vi "Split Start Delays.vi"(0 "Start Delay":dbl, 5 "Value":dbl, 7 "Sequence Delta (s)":dbl) -> (4 "Start Delay":dbl[](array[numeric]), 6 "Value":dbl[](array[numeric]))   [LabVIEW 2024, in "devicePowerSequencerCoreLogic.lvlib"]
uses:
  devicePowerSequencerCoreLogic.lvlib
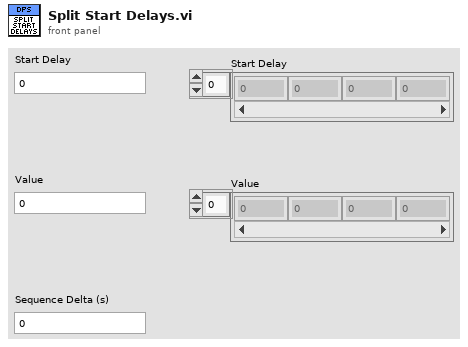
[diagram p1: front panel]
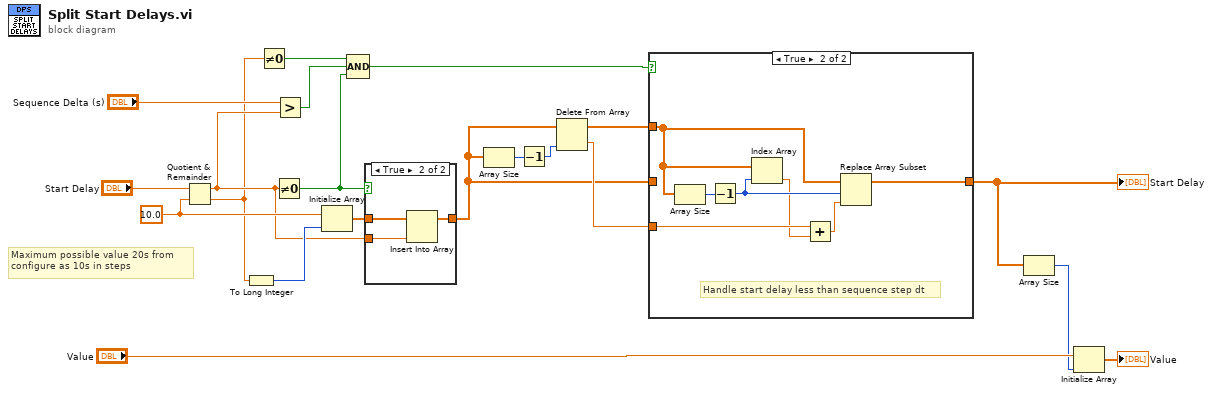
[diagram p0: block diagram]
diagram:
  w20 = 10.0 ("y")
  # "Maximum possible value 20s from\nconfigure as 10s in steps"
  n1 = Quotient & Remainder(x="Start Delay", y=w20) -> (x-y*floor(x/y)=w6:dbl, floor(x/y)=w5:dbl)
  n2 = To Long Integer(number=w5) -> (32bit integer=w18:i32)
  n3 = Not Equal To 0?(x=w5) -> (x != 0?=w4:bool)
  n4 = Not Equal To 0?(x=w6) -> (x != 0?=w2:bool)
  n5 = Greater?(x="Sequence Delta (s)", y=w6) -> (0:w3:bool)
  n6 = Initialize Array(w20, w18) -> (w19:dbl[])
  n7 = Compound Arithmetic op=AND(w4, w3, w2) -> (w1:bool)
  n8 = case shown="True" w2 {
    tunnel: w19 -> [w21 w24]
    tunnel: [w21 w22] -> w9
    tunnel: w6 -> [_ w23]
    frame False {
    }
    frame True {
      n9 = Insert Into Array(array=w24, new element=w23) -> (w22:dbl[])  [unwired: 1 in]
    }
  }
  n10 = Array Size(array=w9) -> (size(s)=w16:i32)
  n11 = Decrement(x=w16) -> (x-1=w15:i32)
  n12 = Delete From Array(array=w9, index=w15) -> (deleted portion=w13:dbl, array with subset deleted=w12:dbl[])  [unwired: 1 in]
  n13 = case shown="True" w1 {
    tunnel: w13 -> [_ w31]
    tunnel: [w25 w29] -> w8
    tunnel: w12 -> [_ w27]
    tunnel: w9 -> [w25 _]
    frame False {
    }
    frame True {
      # "Handle start delay less than sequence step dt"
      n14 = Array Size(array=w27) -> (size(s)=w32:i32)
      n15 = Decrement(x=w32) -> (x-1=w28:i32)
      n16 = Index Array(array=w27, index=w28) -> (element=w26:dbl)
      n17 = Add(x=w31, y=w26) -> (x+y=w30:dbl)
      n18 = Replace Array Subset(array=w27, new element=w30, index=w28) -> (w29:dbl[])
    }
  }
  "Start Delay" <- w8
  n19 = Array Size(array=w8) -> (size(s)=w7:i32)
  n20 = Initialize Array("Value", w7) -> (→"Value":dbl[])
